vi "Galala cPID.vi"() -> ()   [LabVIEW 2021]
uses:
  <vilib>/addons/control/pid/pid.llb/PID (DBL).vi
  <vilib>/addons/control/pid/NI_PID_pid.lvlib
panel:
  in  "output range":cluster{"output high":dbl, "output low":dbl}={"output high"=100.0, "output low"=-100.0} {"output low" format="%.2f"; "output high" format="%.2f"}
  in  "PID gains":T1={"proportional gain (Kc)"=1.0, "integral time (Ti, min)"=0.01, "derivative time (Td, min)"=0.0} {"derivative time (Td, min)" format="%.3f"; "integral time (Ti, min)" format="%.3f"; "proportional gain (Kc)" format="%.3f"}
  in  "setpoint":dbl format="%.2f"
  out "Graph":waveform(dbl)[](graph)
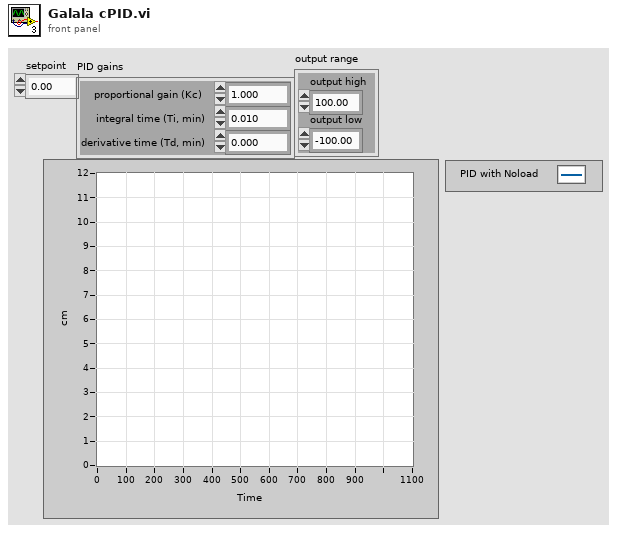
[diagram p1: front panel]
types:
  T1 = cluster{"proportional gain (Kc)":dbl, "integral time (Ti, min)":dbl, "derivative time (Td, min)":dbl}
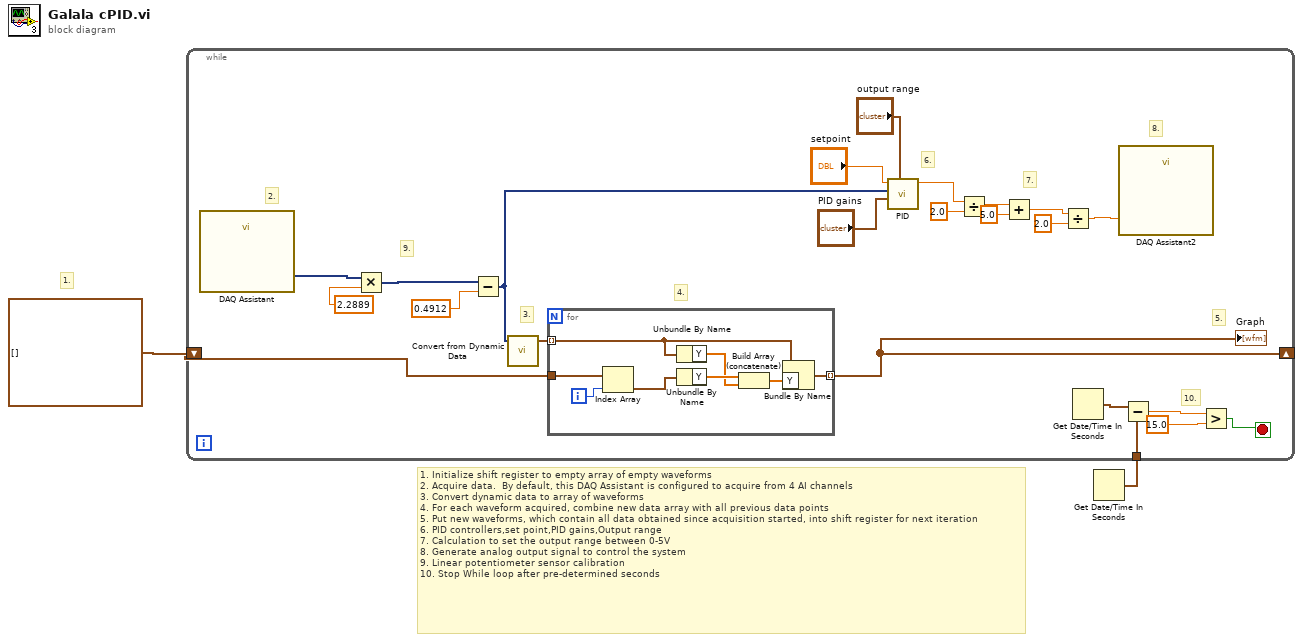
[diagram p0: block diagram]
diagram:
  # "1. Initialize shift register to empty array of empty waveforms\n2. Acquire data.  By default, this DAQ Assistant is configured to acquire from 4 AI channels\n3. Convert dynamic data to array of waveforms\n4. For each waveform acquired, combine new data array with all previous data points\n5. Put new waveforms, which contain all data obtained since acquisition started, into shift register for next iteration\n6. PID controllers,set point,PID gains,Output range\n7. Calculation to set the output range between 0-5V \n8. Generate analog output signal to control the system\n9. Linear potentiometer sensor calibration\n10. Stop While loop after pre-determined seconds"
  # "1."
  n1 = Get Date/Time In Seconds() -> (seconds since 1Jan1904=w1:timestamp)
  n2 = while {
    shift-right: [w18] -> _
    shift-left: waveform(dbl)[] [] -> [w19]
    tunnel: w1 -> [w21]
    stop <- w20 stop-if-true
    # "7."
    # "10."
    # "9."
    # "8."
    # "6."
    # "3."
    # "2."
    # "5."
    # "4."
    n3 = call "DAQ Assistant"() -> ("data"=w12:dynamicdata)  [unwired: 17 in, 2 out]
    n4 = Multiply(x=w12, y=2.2889) -> (x*y=w15:dynamicdata)
    n5 = Subtract(x=w15, y=0.4912) -> (x-y=w3:dynamicdata)
    n6 = call "Convert from Dynamic Data"("Dynamic Data Type"=w3) -> ("Array of Waveform"=w25:waveform(dbl)[])  [unwired: 3 in]
    n7 = for {
      tunnel: w25 -> [w32] mode=indexing
      tunnel: [w29] -> w18 mode=indexing
      tunnel: w19 -> [w28]
      i -> [w27]
      n8 = Index Array(array=w28, index=w27) -> (element=w26:waveform(dbl))
      n9 = Unbundle By Name(w32) -> ("Y"=w30:dbl[])
      n10 = Unbundle By Name(w26) -> ("Y"=w33:dbl[])
      n11 = Build Array (concatenate)(w33, w30) -> (w31:dbl[])
      n12 = Bundle By Name(cluster=w32, "Y"=w31) -> (w29:waveform(dbl))
    }
    "Graph" <- w18
    n13 = call-poly <vilib>:"PID.vi"("output range"="output range", "PID gains"="PID gains", "process variable"=w3, "setpoint"="setpoint") -> ("output"=w7:dbl)  [unwired: 6 in, 1 out]
    n14 = Divide(x=w7, y=2.0) -> (x/y=w6:dbl)
    n15 = Add(x=w6, y=5.0) -> (x+y=w5:dbl)
    n16 = Divide(x=w5, y=2.0) -> (x/y=w4:dbl)
    n17 = Get Date/Time In Seconds() -> (seconds since 1Jan1904=w24:timestamp)
    n18 = call "DAQ Assistant2"("data"=w4) -> ()  [unwired: 17 in, 2 out]
    n19 = Subtract(x=w24, y=w21) -> (x-y=w23:dbl)
    n20 = Greater?(x=w23, y=15.0) -> (0:w20:bool)
  }
